vi "FloatingPointEcho.vi"() -> ()   [LabVIEW 2023]
uses:
  <vilib>/Instr/_visa.llb/VISA Configure Serial Port (Instr).vi
panel:
  in  "Blank Button":bool
  in  "VISA resource name":refnum<visa-resource-name>
  in  "Stop Button":bool
  out "Numeric Indicator 2":sgl format="%#_6f"
  in  "Numeric Control":sgl format="%#_6f"
  in  "Send Button":bool
  # "Floating Point Echo"
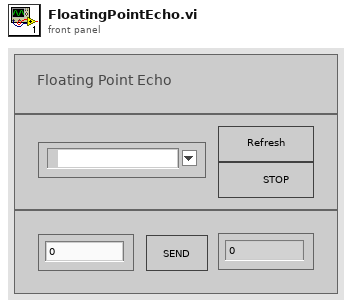
[diagram p1: front panel]
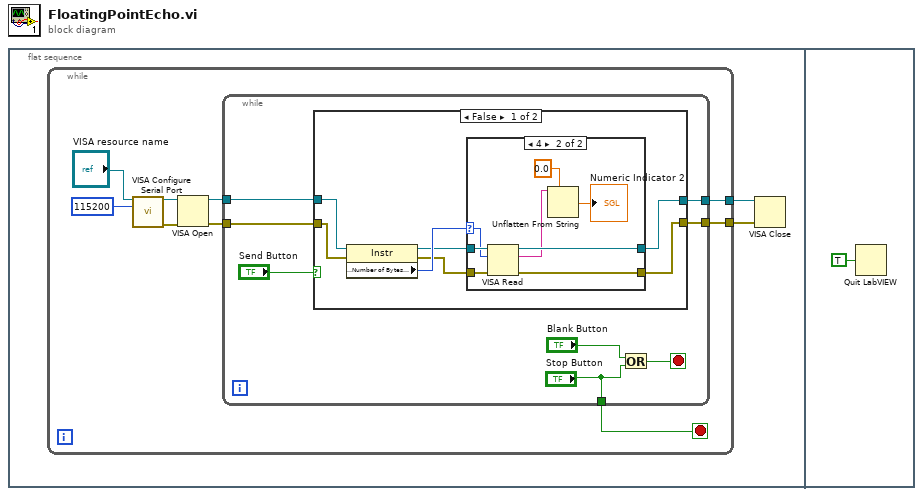
[diagram p0: block diagram]
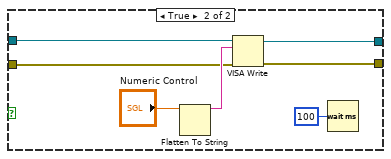
[diagram p3: hidden frame]
diagram:
  n1 = flat-sequence {
    frame #0 {
      n2 = while {
        tunnel: [w5] -> w2
        tunnel: [w4] -> w1
        stop <- w3 stop-if-true
        n3 = call-poly "VISA Configure Serial Port"("VISA resource name"="VISA resource name", "baud rate (9600)"=u32 115200) -> ("VISA resource name out"=w7:refnum<visa-resource-name>, "error out"=w8:errorcluster)  [unwired: 12 in]
        n4 = VISA Open(error in (no error)=w8, VISA resource name=w7) -> (VISA resource name=w9:refnum<visa-resource-name>, error out=w10:errorcluster)  [unwired: 3 in]
        n5 = while {
          tunnel: w9 -> [w16]
          tunnel: w10 -> [w15]
          tunnel: [w18] -> w5
          tunnel: [w17] -> w4
          tunnel: ["Stop Button"] -> w3
          stop <- w12 stop-if-true
          n6 = case shown="False" "Send Button" {
            tunnel: [w21 w41] -> w18
            tunnel: [w20 w40] -> w17
            tunnel: w16 -> [w25 w39]
            tunnel: w15 -> [w24 w38]
            frame False {
              n7 = property class="Instr"(reference=w25, error in=w24) -> (reference out=w23:refnum<visa-resource-name>, error out=w22:errorcluster, "Serial Settings:Number of Bytes at Serial Port"=w26:u32)
              n8 = case shown="4" w26 {
                selector: w26 -> [_ w29]
                tunnel: w23 -> [w28 w34]
                tunnel: w22 -> [w27 w33]
                tunnel: [w28 w32] -> w21
                tunnel: [w27 w31] -> w20
                frame 0, Default {
                }
                frame 4 {
                  n9 = VISA Read(VISA resource name=w34, byte count=w29, error in (no error)=w33) -> (VISA resource name out=w32:refnum<visa-resource-name>, read buffer=w30:string, error out=w31:errorcluster)  [unwired: 1 out]
                  n10 = Unflatten From String(type=sgl 0.0, binary string=w30) -> (value=→"Numeric Indicator 2":sgl)  [unwired: 3 in, 2 out]
                }
              }
            }
            frame True {
              n11 = Flatten To String(anything="Numeric Control") -> (data string=w42:string)  [unwired: 3 in, 2 out]
              n12 = VISA Write(VISA resource name=w39, write buffer=w42, error in (no error)=w38) -> (VISA resource name out=w41:refnum<visa-resource-name>, error out=w40:errorcluster)  [unwired: 1 out]
              n13 = Wait (ms)(milliseconds to wait=u32 100) -> ()  [unwired: 1 out]
            }
          }
          n14 = Or(x="Blank Button", y="Stop Button") -> (x .or. y?=w12:bool)
        }
      }
      n15 = VISA Close(VISA resource name=w2, error in (no error)=w1) -> ()  [unwired: 1 out]
    }
    frame #1 {
      n16 = Quit LabVIEW(quit? (T)=TRUE) -> ()
    }
  }
